vi "test_libssh2_userauth_publickey_frommemory.vi"() -> ()   [LabVIEW 2013, in "libssh2_integration_tests.lvlib"]
uses:
  libssh2_integration_tests.lvlib
  libssh2/libssh2_init_default.vi
  libssh2/libssh2_session_handshake_tcp.vi
  libssh2/libssh2.lvlib
  <vilib>/addons/_JKI Toolkits/Caraya/classes/Test/Test.lvclass
  support/support.lvlib
  <vilib>/addons/_JKI Toolkits/Caraya/classes/Assert/Assert.lvclass
panel:
  out "error out":errorcluster
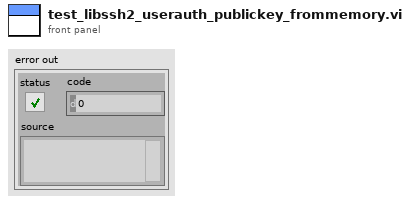
[diagram p1: front panel]
types:
  T1 = typedef "libssh2.lvlib/Session Refnum.ctl" = refnum<k1>
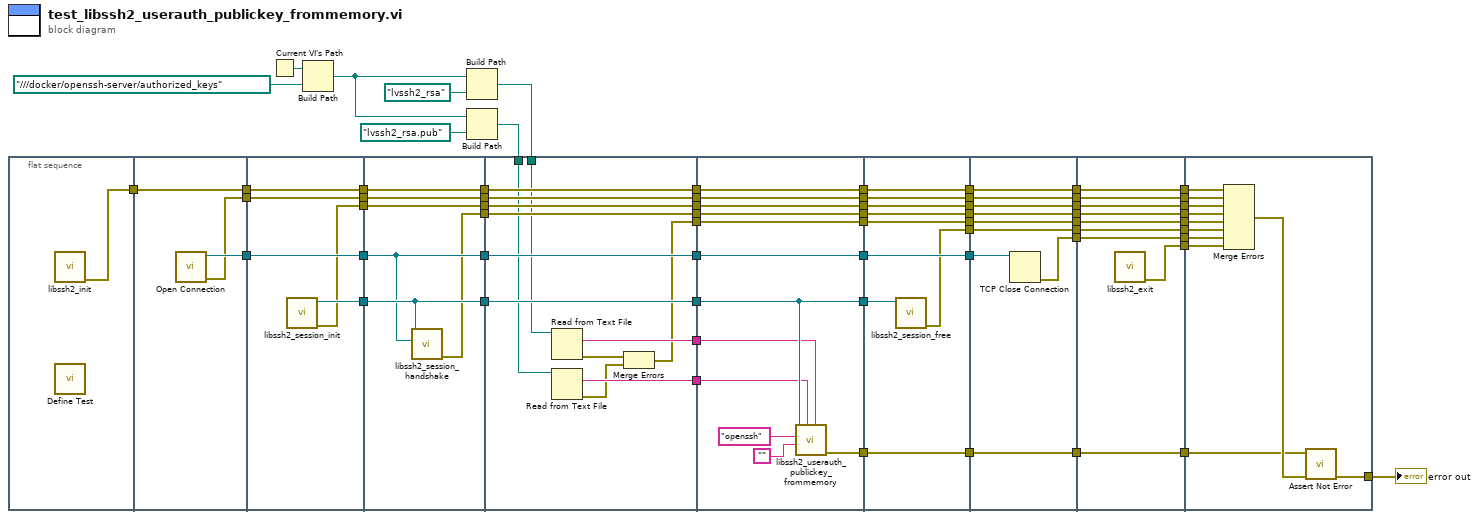
[diagram p0: block diagram]
diagram:
  n1 = flat-sequence {
    tunnel: [w66] -> w65
    tunnel: [w69] -> w64
    tunnel: w65 -> [w68]
    tunnel: [w68] -> w63
    tunnel: [w67] -> w62
    tunnel: w64 -> [w74]
    tunnel: [w74] -> w41
    tunnel: w63 -> [w73]
    tunnel: [w73] -> w40
    tunnel: w62 -> [w72]
    tunnel: [w72] -> w39
    tunnel: [w71] -> w38
    tunnel: [w70] -> w37
    tunnel: w41 -> [w76]
    tunnel: [w76] -> w21
    tunnel: w40 -> [w80]
    tunnel: [w80] -> w19
    tunnel: w39 -> [w79]
    tunnel: [w79] -> w17
    tunnel: [w78] -> w15
    tunnel: w38 -> [w78]
    tunnel: w37 -> [w77]
    tunnel: [w77] -> w13
    tunnel: [w75] -> w11
    tunnel: w21 -> [w93]
    tunnel: [w93] -> w20
    tunnel: w19 -> [w92]
    tunnel: [w92] -> w18
    tunnel: w17 -> [w91]
    tunnel: [w91] -> w16
    tunnel: w15 -> [w90]
    tunnel: [w90] -> w14
    tunnel: w13 -> [w89]
    tunnel: [w89] -> w12
    tunnel: w11 -> [w88]
    tunnel: [w88] -> w10
    tunnel: [w87] -> w9
    tunnel: [w86] -> w8
    tunnel: w7 -> [w85]
    tunnel: w6 -> [w84]
    tunnel: [w81] -> w5
    tunnel: w20 -> [w105]
    tunnel: [w105] -> w33
    tunnel: w18 -> [w104]
    tunnel: [w104] -> w32
    tunnel: w16 -> [w103]
    tunnel: [w103] -> w31
    tunnel: w14 -> [w100]
    tunnel: w12 -> [w102]
    tunnel: [w102] -> w30
    tunnel: w10 -> [w101]
    tunnel: [w101] -> w29
    tunnel: [w100] -> w28
    tunnel: [w98] -> w27
    tunnel: w9 -> [w96]
    tunnel: w8 -> [w95]
    tunnel: w5 -> [w94]
    tunnel: [w94] -> w4
    tunnel: w33 -> [w114]
    tunnel: [w114] -> w50
    tunnel: w32 -> [w113]
    tunnel: [w113] -> w49
    tunnel: w31 -> [w112]
    tunnel: [w112] -> w48
    tunnel: w30 -> [w111]
    tunnel: [w111] -> w47
    tunnel: w29 -> [w110]
    tunnel: [w110] -> w46
    tunnel: [w109] -> w43
    tunnel: [w108] -> w34
    tunnel: w27 -> [w108]
    tunnel: w28 -> [w107]
    tunnel: w4 -> [w106]
    tunnel: [w106] -> w3
    tunnel: w50 -> [w123]
    tunnel: w49 -> [w122]
    tunnel: [w122] -> w61
    tunnel: w48 -> [w121]
    tunnel: [w121] -> w60
    tunnel: [w120] -> w59
    tunnel: w47 -> [w119]
    tunnel: [w119] -> w58
    tunnel: w46 -> [w118]
    tunnel: [w118] -> w57
    tunnel: [w117] -> w44
    tunnel: w43 -> [w117]
    tunnel: [w116] -> w35
    tunnel: w34 -> [w116]
    tunnel: w3 -> [w115]
    tunnel: [w115] -> w2
    tunnel: w61 -> [w132]
    tunnel: [w132] -> w56
    tunnel: w60 -> [w131]
    tunnel: [w131] -> w55
    tunnel: w59 -> [w130]
    tunnel: [w130] -> w54
    tunnel: [w129] -> w53
    tunnel: w58 -> [w128]
    tunnel: [w128] -> w52
    tunnel: w57 -> [w127]
    tunnel: [w127] -> w51
    tunnel: [w126] -> w45
    tunnel: w44 -> [w126]
    tunnel: [w125] -> w36
    tunnel: w35 -> [w125]
    tunnel: w2 -> [w124]
    tunnel: [w124] -> w1
    tunnel: w56 -> [w143]
    tunnel: w55 -> [w142]
    tunnel: w54 -> [w141]
    tunnel: w53 -> [w140]
    tunnel: w52 -> [w139]
    tunnel: [w137] -> w42
    tunnel: w51 -> [w136]
    tunnel: w45 -> [w135]
    tunnel: w36 -> [w134]
    tunnel: w1 -> [w133]
    frame #0 {
      n2 = call-poly "libssh2_init.vi"() -> ("error out"=w66:errorcluster)  [unwired: 11 in]
      n3 = call <vilib>:"Define Test.vi"() -> ()  [unwired: 10 in, 2 out]
    }
    frame #1 {
      n4 = call "Open Connection.vi"() -> ("error out"=w67:errorcluster, "connection ID"=w69:refnum<k5>)  [unwired: 10 in]
    }
    frame #2 {
      n5 = call "libssh2_session_init.vi"() -> ("error out"=w70:errorcluster, "session"=w71:T1)  [unwired: 10 in]
    }
    frame #3 {
      n6 = call-poly "libssh2_session_handshake.vi"("tcp connection"=w76, "session"=w78) -> ("error out"=w75:errorcluster)  [unwired: 9 in]
    }
    frame #4 {
      n7 = Read from Text File(file (use dialog)=w85) -> (text=w86:string, error out=w82:errorcluster)  [unwired: 3 in, 2 out]
      n8 = Read from Text File(file (use dialog)=w84) -> (text=w87:string, error out=w83:errorcluster)  [unwired: 3 in, 2 out]
      n9 = Merge Errors(w82, w83) -> (w81:errorcluster)
    }
    frame #5 {
      n10 = call "libssh2_userauth_publickey_frommemory.vi"("private key data"=w95, "public key data"=w96, "passphrase"="", "username"="openssh", "session"=w100) -> ("error out"=w98:errorcluster)  [unwired: 6 in]
    }
    frame #6 {
      n11 = call "libssh2_session_free.vi"("session"=w107) -> ("error out"=w109:errorcluster)  [unwired: 10 in]
    }
    frame #7 {
      n12 = TCP Close Connection(connection ID=w123) -> (error out=w120:errorcluster)  [unwired: 2 in, 1 out]
    }
    frame #8 {
      n13 = call "libssh2_exit.vi"() -> ("error out"=w129:errorcluster)  [unwired: 11 in]
    }
    frame #9 {
      n14 = Merge Errors(w143, w142, w139, w136, w133, w135, w141, w140) -> (w138:errorcluster)
      n15 = call <vilib>:"Assert Not Error.vi"("error in (no error)"=w138, "Not Error?"=w134) -> ("error out"=w137:errorcluster)  [unwired: 8 in, 1 out]
    }
  }
  n16 = Current VI's Path() -> (path=w22:path)
  n17 = Build Path(base path=w22, name or relative path=path "../../../docker/openssh-server/authorized_keys" ("stripped path")) -> (appended path=w23:path)
  n18 = Build Path(base path=w23, name or relative path=path "lvssh2_rsa" ("stripped path")) -> (appended path=w7:path)
  n19 = Build Path(base path=w23, name or relative path=path "lvssh2_rsa.pub" ("stripped path")) -> (appended path=w6:path)
  "error out" <- w42
